vi "hpcnc wait idle.vi"(10 "error in (no error)":errorcluster, 11 "VISA Refnum in":refnum<visa-resource-name>) -> (0 "error out":errorcluster, 1 "VISA Refnum out":refnum<visa-resource-name>, 3 "Idle":bool)   [LabVIEW 2014]
uses:
  HPCNC.lvlib
panel:
  out "error in (no error) 2":errorcluster
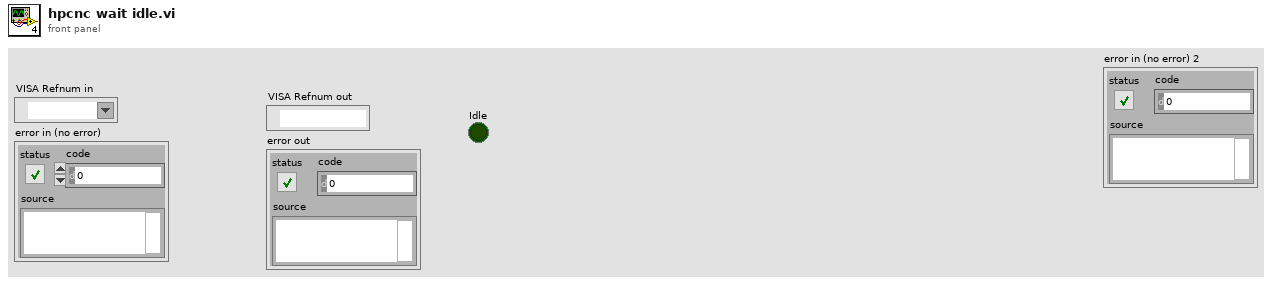
[diagram p1: front panel]
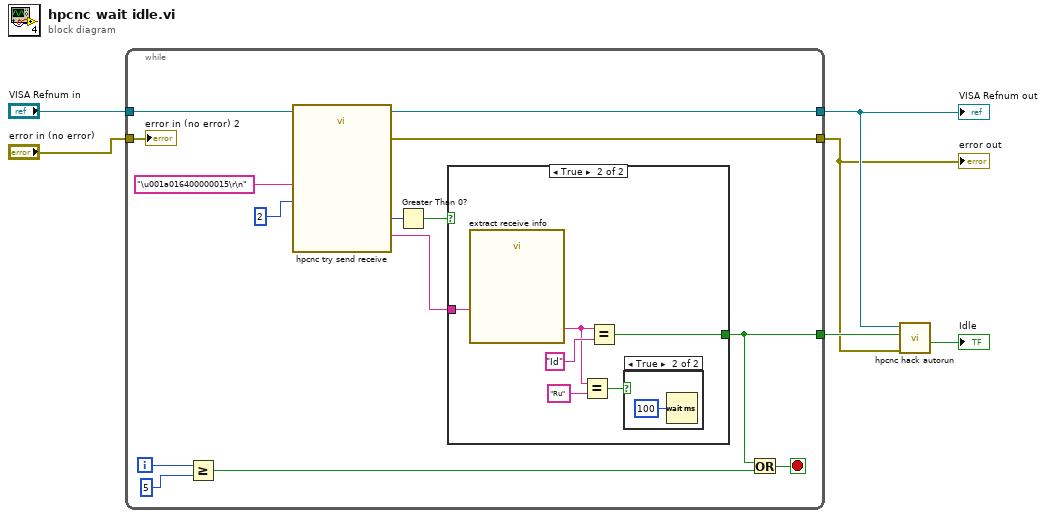
[diagram p0: block diagram]
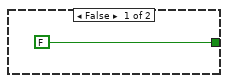
[diagram p2: hidden frame]
diagram:
  n1 = while {
    tunnel: "VISA Refnum in" -> [w17]
    tunnel: "error in (no error)" -> [w7]
    tunnel: [w14] -> w2
    tunnel: [w13] -> w1
    tunnel: [w8] -> w4
    i -> [w9]
    stop <- w11 stop-if-true
    n2 = Greater Or Equal?(x=w9, y=5) -> (x >= y?=w18:bool)
    n3 = call "hpcnc try send receive.vi"("Max try number"=2, "Send package"="\u001a016400000015\r\n" ("SendData"), "VISA Refnum in"=w17) -> ("error out"=w13:errorcluster, "Receive count"=w15:i32, "Receive package"=w12:string, "VISA Refnum out"=w14:refnum<visa-resource-name>)  [unwired: 5 in]
    n4 = Greater Than 0?(x=w15) -> (x > 0?=w16:bool)
    n5 = case shown="True" w16 {
      tunnel: w12 -> [_ w26]
      tunnel: [FALSE w25] -> w8
      frame False {
      }
      frame True {
        n6 = call "extract receive info.vi"("Receive data"=w26) -> ("STATUS"=w24:string)  [unwired: 11 in, 3 out]
        n7 = Equal?(x=w24, y="Ru") -> (x = y?=w22:bool)
        n8 = Equal?(x=w24, y="Id") -> (x = y?=w25:bool)
        n9 = case shown="True" w22 {
          frame False {
          }
          frame True {
            n10 = Wait (ms)(milliseconds to wait=u32 100) -> ()  [unwired: 1 out]
          }
        }
      }
    }
    n11 = Or(x=w8, y=w18) -> (x .or. y?=w11:bool)
    "error in (no error) 2" <- w7
  }
  "VISA Refnum out" <- w2
  "error out" <- w1
  n12 = call "hpcnc hack autorun.vi"("error in (no error)"=w1, "Idle"=w4, "VISA Refnum in"=w2) -> ("Reset"=→"Idle":bool)  [unwired: 7 in]
